vi "Run.vi"(7 "Team Index":i32, 8 "Column":i32, 9 "Row":i32, 10 "View":i32[](array[numeric]) caption="View (Team Index, -1: empty)", 11 "Tim_The_Enchanter In":refnum<class "Tim_The_Enchanter.lvclass">) -> (0 "Replicated":refnum<class "Square.lvclass">, 1 "Direction":T1, 2 "Action":T2, 3 "Square Out":refnum<class "Square.lvclass">)   [LabVIEW 2016, in "Tim_The_Enchanter.lvclass"]
uses:
  Tim_The_Enchanter.lvclass
  C:/Users/Events/Desktop/SquareBattle/Square/Square.lvclass
  Square/Square.lvclass
  Type Defs/Action Enum.ctl
  Type Defs/Direction Enum.ctl
  SubVIs/Read-Only Globals.vi
  SubVIs/Globals (private).vi
  Common/Common.lvlib
  Type Defs/SB Type Defs.lvlib
panel:
  # "NW\nN\nNE\nE\nSE\nS\nSW\nW"
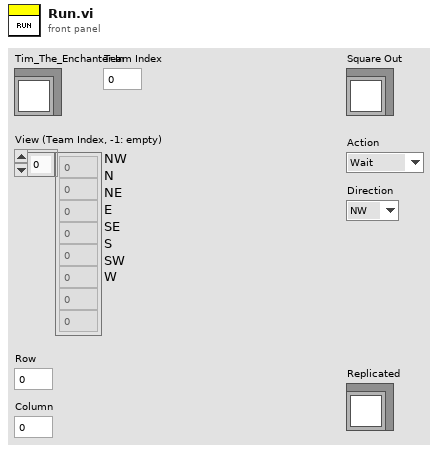
[diagram p1: front panel]
types:
  T1 = typedef "SB Type Defs.lvlib/Direction Enum.ctl" = enum16{"NW", "N", "NE", "E", "SE", "S", "SW", "W"}
  T2 = typedef "SB Type Defs.lvlib/Action Enum.ctl" = enum16{"Wait", "Move", "Attack", "Replicate"}
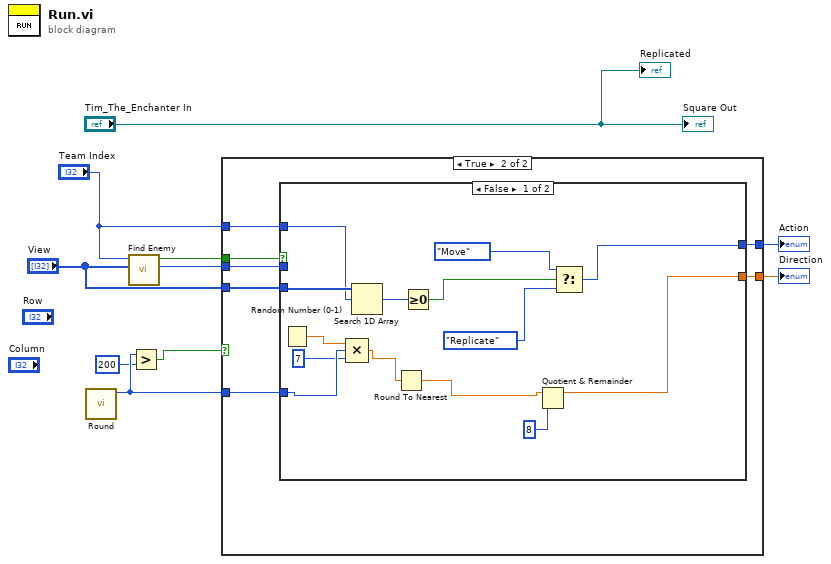
[diagram p0: block diagram]
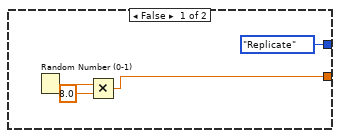
[diagram p2: hidden frame]
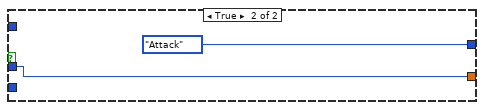
[diagram p3: hidden frame]
diagram:
  n1 = call "Round.vi"() -> ("Round"=w3:i32)  [unwired: 11 in]
  n2 = call "Find Enemy.vi"("View"="View", "Team Index"="Team Index") -> ("Direction"=w8:T1, "Found Enemy?"=w9:bool)  [unwired: 7 in, 1 out]
  n3 = Greater?(x=w3, y=200) -> (0:w1:bool)
  n4 = case shown="True" w1 {
    tunnel: w9 -> [_ w21]
    tunnel: w8 -> [_ w20]
    tunnel: [Action_Enum."Replicate" ("Action") w19] -> w7
    tunnel: "View" -> [_ w18]
    tunnel: "Team Index" -> [_ w17]
    tunnel: w3 -> [_ w16]
    tunnel: [w11 w15] -> w4
    frame False {
      n5 = Random Number (0-1)() -> (number: 0 to 1=w13:dbl)
      n6 = Multiply(x=w13, y=8.0) -> (x*y=w11:dbl)
    }
    frame True {
      n7 = case shown="False" w21 {
        tunnel: w20 -> [_ w36]
        tunnel: [w29 Action_Enum."Attack" ("Action")] -> w19
        tunnel: w18 -> [w35 _]
        tunnel: w17 -> [w34 _]
        tunnel: w16 -> [w26 _]
        tunnel: [w22 w36] -> w15
        frame False {
          n8 = Random Number (0-1)() -> (number: 0 to 1=w27:dbl)
          n9 = Compound Arithmetic op=MULTIPLY(w27, w26, 7 ("value")) -> (w24:dbl)
          n10 = Search 1D Array(1D array=w35, element=w34) -> (index of element=w33:i32)  [unwired: 1 in]
          n11 = Round To Nearest(number=w24) -> (nearest integer value=w23:dbl)
          n12 = Greater Or Equal To 0?(x=w33) -> (x >= 0?=w30:bool)
          n13 = Quotient & Remainder(x=w23, y=8) -> (x-y*floor(x/y)=w22:dbl)  [unwired: 1 out]
          n14 = Select(t=Action_Enum."Move" ("Action"), s=w30, f=Action_Enum."Replicate" ("Action")) -> (s? t:f=w29:T2)
        }
        frame True {
        }
      }
    }
  }
  "Action" <- w7
  "Direction" <- w4
  "Square Out" <- "Tim_The_Enchanter In"
  "Replicated" <- "Tim_The_Enchanter In"
